vi "StringToNode(viaString).vi"(0 "Tree DVR in":refnum<data-value>, 1 "String value in":string, 3 "error in (no error)":errorcluster, 4 "NodePath":string) -> (7 "error out":errorcluster)   [LabVIEW 2014]
uses:
  <vilib>/MDSplus/Classes/Tree_Class/Tree.lvclass
  <vilib>/MDSplus/Library/MDSplus.lvlib
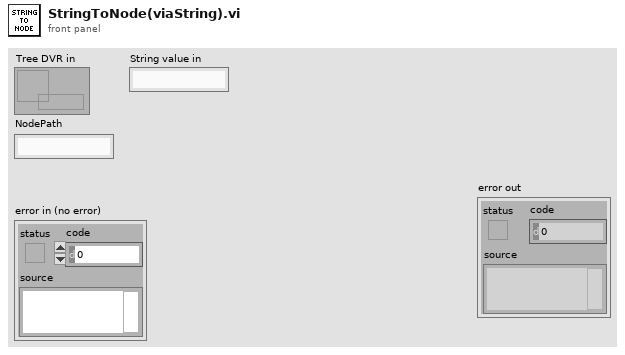
[diagram p1: front panel]
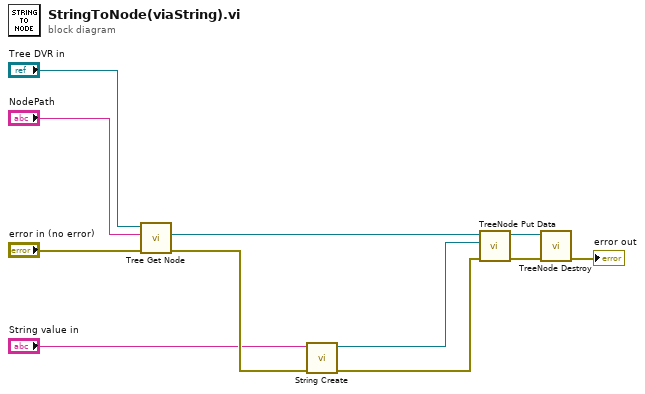
[diagram p0: block diagram]
diagram:
  n1 = call <vilib>:"Tree Get Node.vi"("error in (no error)"="error in (no error)", "Path"="NodePath", "Tree DVR in"="Tree DVR in") -> ("error out"=w7:errorcluster, "Node out"=w4:refnum<data-value>)  [unwired: 6 in, 1 out]
  n2 = call <vilib>:"String Create.vi"("error in (no error)"=w7, "String value in"="String value in") -> ("error out"=w8:errorcluster, "String DVR out"=w5:refnum<data-value>)  [unwired: 8 in]
  n3 = call <vilib>:"TreeNode Put Data.vi"("error in (no error)"=w8, "Data"=w5, "TreeNode DVR in"=w4) -> ("error out"=w2:errorcluster, "TreeNode DVR out"=w3:refnum<data-value>)  [unwired: 7 in]
  n4 = call <vilib>:"TreeNode Destroy.vi"("error in (no error)"=w2, "TreeNode DVR in"=w3) -> ("error out"=→"error out":errorcluster)  [unwired: 9 in]
